vi "raptor_getlag.vi"(8 "error in (no error)":errorcluster) -> (0 "error out":errorcluster, 3 "Frame Lag":i32)   [LabVIEW 2016]
doc: "Raptor: Returns number of frames to be processed in queue."
uses:
  typedef/raptor_image.ctl
  <vilib>/vision/Image Controls.llb/IMAQ Image.ctl
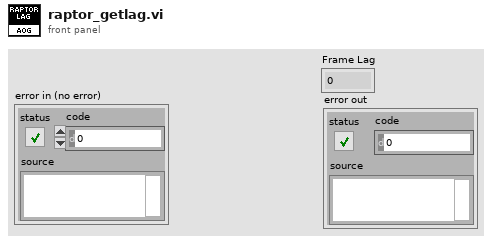
[diagram p1: front panel]
types:
  T1 = typedef "raptor_image.ctl" = cluster{"Data":variant, "Image":T2}
  T2 = typedef "IMAQ Image.ctl" = refnum<image>
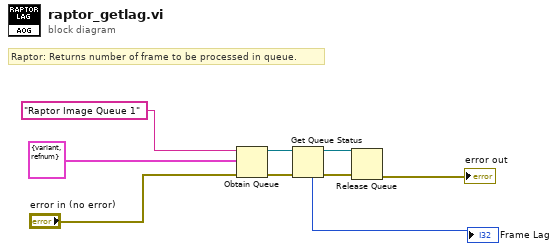
[diagram p0: block diagram]
diagram:
  # "Raptor: Returns number of frame to be processed in queue."
  n1 = Obtain Queue(name (unnamed)="Raptor Image Queue 1", element data type=T1 {"Data"=variant, "Image"=refnum} ("Cluster"), error in (no error)="error in (no error)") -> (queue out=w8:refnum<queue>, error out=w4:errorcluster)  [unwired: 2 in, 1 out]
  n2 = Get Queue Status(queue=w8, error in (no error)=w4) -> (queue out=w2:refnum<queue>, error out=w3:errorcluster, # elements in queue=→"Frame Lag":i32)  [unwired: 1 in, 5 out]
  n3 = Release Queue(queue=w2, error in (no error)=w3) -> (error out=→"error out":errorcluster)  [unwired: 1 in, 2 out]
